vi "enterIntoHierarchy.vi"(8 "error in (no error)":errorcluster, 10 "output array of keys":string[](array[string]), 11 "Variant in":variant) -> (0 "error out":errorcluster, 3 "Variant out":variant)   [LabVIEW 2015, in "Zen Analytics.lvclass"]
uses:
  Zen Analytics.lvclass
  <vilib>/regexp/Match Regular Expression.xnode
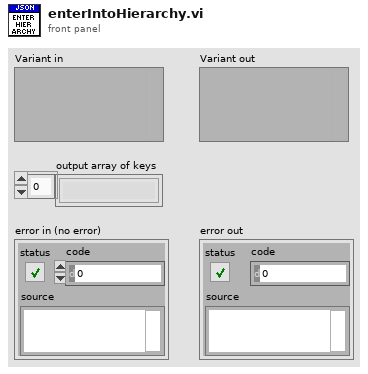
[diagram p1: front panel]
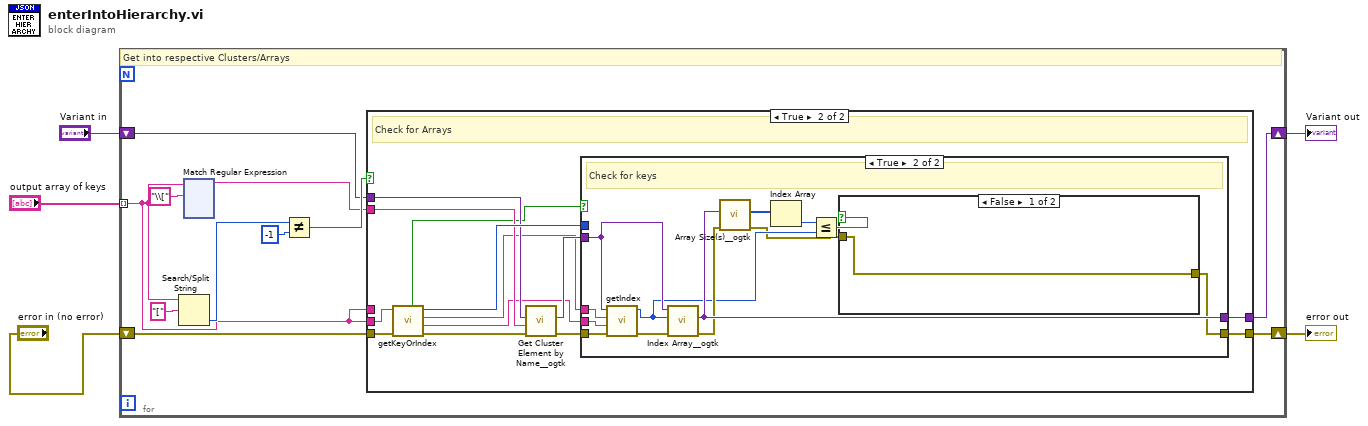
[diagram p0: block diagram]
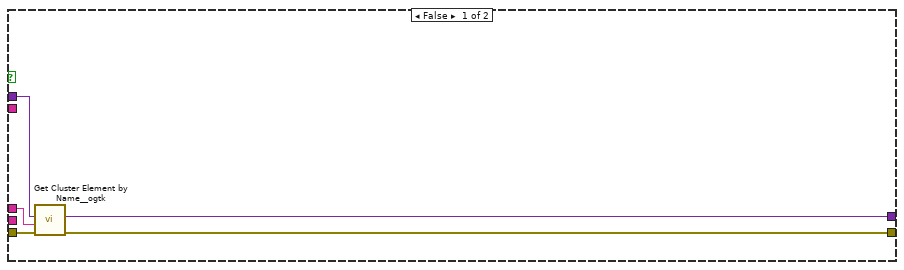
[diagram p2: hidden frame]
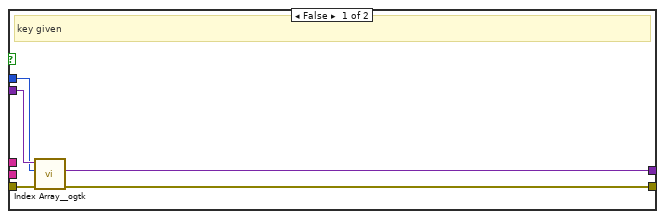
[diagram p3: hidden frame]
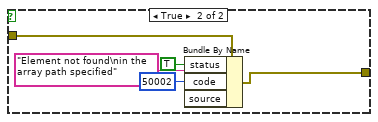
[diagram p4: hidden frame]
diagram:
  n1 = for {
    tunnel: "output array of keys" -> [w6] mode=indexing
    shift-right: [w13] -> w4
    shift-left: "Variant in" -> [w14]
    shift-right: [w11] -> w5
    shift-left: "error in (no error)" -> [w12]
    # "Get into respective Clusters/Arrays"
    n2 = Search/Split String(string=w6, search string/char (-)="[") -> (offset of match=w7:i32)  [unwired: 1 in, 2 out]
    n3 = xnode "Match Regular Expression"("input string"=w6, "regular expression"="\\[") -> ("before match"=w9:string)  [unwired: 4 in, 4 out]
    n4 = Not Equal?(x=w7, y=-1) -> (x != y?=w15:bool)
    n5 = case shown="True" w15 {
      tunnel: w6 -> [_ w146]
      tunnel: w14 -> [w135 w144]
      tunnel: [w133 w148] -> w13
      tunnel: w6 -> [w134 _]
      tunnel: w12 -> [w132 w140]
      tunnel: [w131 w147] -> w11
      tunnel: w9 -> [_ w142]
      frame False {
        n6 = call <userlib>:"Get Cluster Element by Name__ogtk.vi"("error in (no error)"=w132, "Element Name"=w134, "Cluster"=w135) -> ("error out"=w131:errorcluster, "VElement"=w133:variant)  [unwired: 6 in, 1 out]
      }
      frame True {
        # "Check for Arrays"
        n7 = call "getKeyOrIndex.vi"("error in (no error)"=w140, "input string"=w146) -> ("error out"=w139:errorcluster, "value"=w137:string, "key"=w138:string, "index"=w145:i32, "keygiven?"=w136:bool)  [unwired: 5 in]
        n8 = call <userlib>:"Get Cluster Element by Name__ogtk.vi"("error in (no error)"=w139, "Element Name"=w142, "Cluster"=w144) -> ("error out"=w141:errorcluster, "VElement"=w143:variant)  [unwired: 6 in, 1 out]
        n9 = case shown="True" w136 {
          tunnel: [w153 w161] -> w148
          tunnel: [w152 w154] -> w147
          tunnel: w143 -> [w151 w163]
          tunnel: w141 -> [w150 w165]
          tunnel: w145 -> [w149 _]
          tunnel: w138 -> [_ w166]
          tunnel: w137 -> [_ w164]
          frame False {
            # "key given"
            n10 = call <userlib>:"Index Array__ogtk.vi"("error in (no error)"=w150, "Index (1D)"=w149, "MultiD Array"=w151) -> ("error out"=w152:errorcluster, "Array Element"=w153:variant)  [unwired: 7 in]
          }
          frame True {
            # "Check for keys"
            n11 = call "getIndex.vi"("error in (no error)"=w165, "value"=w164, "key"=w166, "VElement"=w163) -> ("error out"=w162:errorcluster, "indexOut"=w157:i32)  [unwired: 6 in]
            n12 = call <userlib>:"Index Array__ogtk.vi"("error in (no error)"=w162, "Index (1D)"=w157, "MultiD Array"=w163) -> ("error out"=w160:errorcluster, "Array Element"=w161:variant)  [unwired: 7 in]
            n13 = call <userlib>:"Array Size(s)__ogtk.vi"("error in (no error)"=w160, "Array"=w161) -> ("error out"=w155:errorcluster, "Size(s)"=w159:u32[])  [unwired: 7 in, 1 out]
            n14 = Index Array(array=w159) -> (element=w158:u32)  [unwired: 1 in]
            n15 = Less Or Equal?(x=w158, y=w157) -> (x <= y?=w156:bool)
            n16 = case shown="False" w156 {
              tunnel: w155 -> [w167 w172]
              tunnel: [w167 w168] -> w154
              frame False {
              }
              frame True {
                n17 = Bundle By Name(cluster=w172, "status"=TRUE, "code"=50002, "source"="Element not found\nin the array path specified") -> (w168:errorcluster)
              }
            }
          }
        }
      }
    }
  }
  "error out" <- w5
  "Variant out" <- w4
